vi "Actor Destroy.vi"(11 "Self Actor in":refnum<class "Self Actor.lvclass">) -> (0 "error out":errorcluster, 3 "Self Actor out":refnum<class "Self Actor.lvclass">)   [LabVIEW 2021, in "jettl.lvlib" / "Self Actor.lvclass"]
uses:
  Self Actor.lvclass
  C:/git/jettl/src/LVCAM/LVCAM/Actor/Actor.lvclass
  Destroying Self Actor State/Destroying Self Actor State.lvclass
  C:/git/jettl/src/LVCAM/LVCAM/Self Actor State/Self Actor State.lvclass
  Self Actor.lvclass/Self Actor.ctl
  Self Actor State/Self Actor State.lvclass
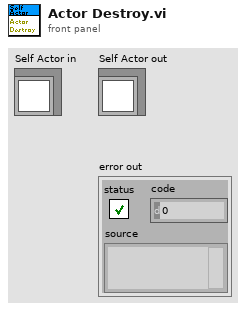
[diagram p1: front panel]
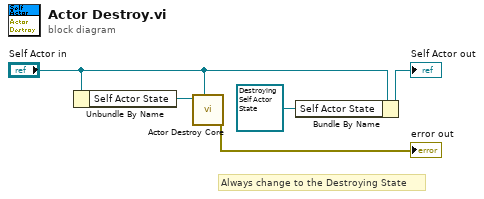
[diagram p0: block diagram]
diagram:
  # "Always change to the Destroying State"
  n1 = Unbundle By Name("Self Actor in") -> ("Self Actor State"=w4:refnum<class "Self Actor State.lvclass">)
  n2 = call-dynamic "Actor Destroy Core.vi"("Actor"="Self Actor in", "Self Actor State in"=w4) -> ("error out"=→"error out":errorcluster)  [unwired: 9 in]
  n3 = Bundle By Name(cluster="Self Actor in", "Self Actor State"=refnum<class "Destroying Self Actor State.lvclass"> refnum ("LVCAM.lvlib:Destroying Self Actor State.lvclass")) -> (→"Self Actor out":refnum<class "Self Actor.lvclass">)
